vi "FlatToRichnidevice_grpc_DeviceProperties.vi"(5 "OutputClusterType":T1, 11 "InputCluster":T2) -> (3 "OutputCluster":T1)   [LabVIEW 2021, in "NI DAQmx_server.lvlib"]
uses:
  NI DAQmx_server.lvlib
  nidevice_grpc_DeviceProperties_Flat.ctl
  nidevice_grpc_DeviceProperties.ctl
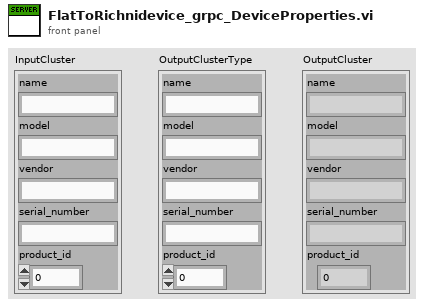
[diagram p1: front panel]
types:
  T1 = typedef "NI DAQmx_server.lvlib/nidevice_grpc_DeviceProperties.ctl" = cluster{"name":string, "model":string, "vendor":string, "serial_number":string, "product_id":u32}
  T2 = typedef "NI DAQmx_server.lvlib/nidevice_grpc_DeviceProperties_Flat.ctl" = cluster{"name":string, "model":string, "vendor":string, "serial_number":string, "product_id":u32}
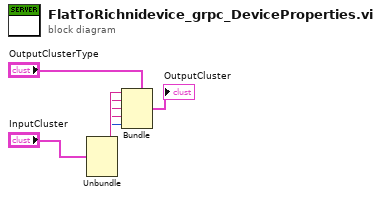
[diagram p0: block diagram]
diagram:
  n1 = Unbundle "Unbundle"("InputCluster") -> ("name"=w5:string, "model"=w4:string, "vendor"=w3:string, "serial_number"=w2:string, "product_id"=w1:u32)
  n2 = Bundle "Bundle"(cluster="OutputClusterType", "name"=w5, "model"=w4, "vendor"=w3, "serial_number"=w2, "product_id"=w1) -> (→"OutputCluster":T1)
